vi "Begin.vi"(8 "error in":errorcluster) -> (0 "error out":errorcluster)   [LabVIEW 2015]
doc: "Called before other user functions, this VI is expected to open initial I/O refnums, load in file data, and do all program initialization. Notice that the <B>error out</B> terminal is simply used for data flow. Wiring it to other structures or subVIs ensures that this VI runs first."
uses:
  <vilib>/Rock Robotics/WPI/DriverStation/WPI_DriverStationRobotMode2.ctl
  <vilib>/Rock Robotics/WPI/Joystick/WPI_JoystickDeviceEnum.ctl
  <vilib>/Rock Robotics/SystemInterfaces/DIO/FPGA_DIOPWMChannel.ctl
  <vilib>/Rock Robotics/WPI/SafetyOutput/WPI_SafetyOutputConfigMenu.ctl
  <vilib>/Rock Robotics/SystemInterfaces/DIO/FPGA_DIOChannel.ctl
  <vilib>/Rock Robotics/WPI/Encoder/WPI_EncoderType.ctl
  <vilib>/Rock Robotics/WPI/CAN/TalonSRX/WPI_CANTalonSRX_APIControlMode.ctl
  <vilib>/Rock Robotics/WPI/CAN/TalonSRX/WPI_CANTalonSRX_APIFeedbackSelect.ctl
  Robot Global Data.vi
  <vilib>/Rock Robotics/Network Tables/NT Write String Array.vi
  <vilib>/Rock Robotics/WPI/RobotDrive/WPI_RobotDriveOpen2MotorWithTalon.vi
  <vilib>/Rock Robotics/WPI/Counter/WPI_CounterDigitalInputToDigitalSource.vi
  <vilib>/Rock Robotics/WPI/MotorControl/WPI_MotorControlOpenCANTalonSRX.vi
  <vilib>/Rock Robotics/WPI/RobotDrive/WPI_RobotDriveOpen2MotorWithJaguar.vi
panel:
  in  "I":dbl
  in  "F":dbl=0.01
  in  "D":dbl
  in  "P":dbl=1.0
  in  "Reverse Feedback Sensor":bool
  in  "Slave Device Number":u8=1
  in  "Encoder Codes Per Rev":u16=360
  in  "Master Device Number":u8
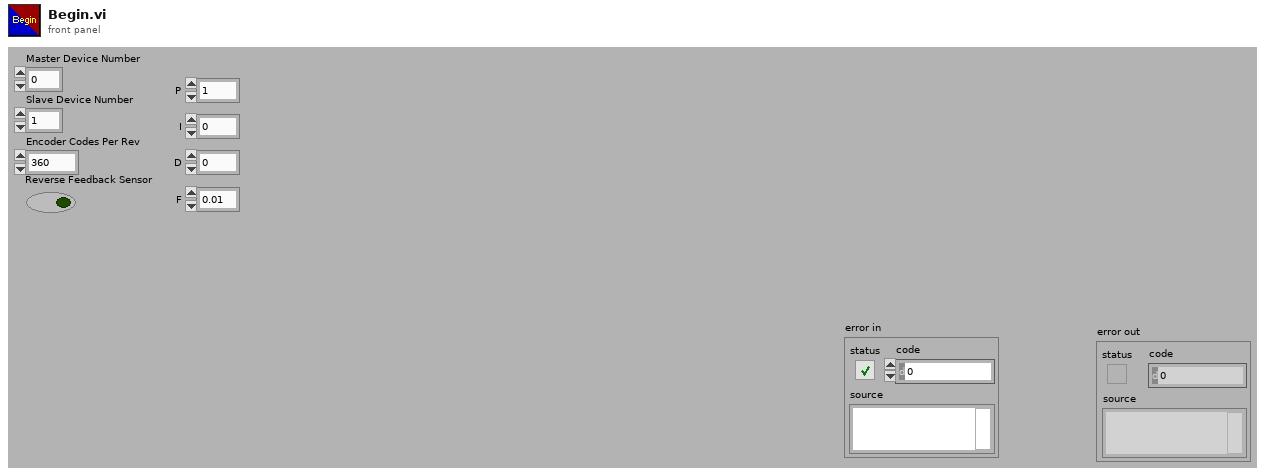
[diagram p1: front panel]
types:
  T1 = typedef "WPI_CANTalonSRX_APIControlMode.ctl" = enum8{"Percent VBus", "Speed", "Position", "Slave", "Unchanged / Invalid", "Voltage Compensation", "Current", "Motion Profile"}
  T2 = typedef "WPI_CANTalonSRX_APIFeedbackSelect.ctl" = enum16{"Digital Quadrature Encoder", "Analog Potentiometer", "Analog Encoder", "Count on Quad-A (Rising-Edge)", "Count on Quad-A (Falling-Edge)", "CTR Magnetic Enc (Absolute)", "CTR Magnetic Enc (Relative)", "Pulse Width"}
  T3 = typedef "WPI_EncoderType.ctl" = enum16{"1x", "2x", "4x"}
  T4 = typedef "FPGA_DIOChannel.ctl" = enum8{"DIO 0", "DIO 1", "DIO 2", "DIO 3", "DIO 4", "DIO 5", "DIO 6", "DIO 7", "DIO 8", "DIO 9", "DIO MXP 0", "DIO MXP 1", "DIO MXP 2", "DIO MXP 3", "DIO MXP 4", "DIO MXP 5", "DIO MXP 6", "DIO MXP 7", "DIO MXP 8", "DIO MXP 9", "DIO MXP 10", "DIO MXP 11", "DIO MXP 12", "DIO MXP 13", "DIO MXP 14", "DIO MXP 15", "Invalid"}
  T5 = typedef "FPGA_DIOPWMChannel.ctl" = enum8{"PWM 0", "PWM 1", "PWM 2", "PWM 3", "PWM 4", "PWM 5", "PWM 6", "PWM 7", "PWM 8", "PWM 9", "PWM MXP 0", "PWM MXP 1", "PWM MXP 2", "PWM MXP 3", "PWM MXP 4", "PWM MXP 5", "PWM MXP 6", "PWM MXP 7", "PWM MXP 8", "PWM MXP 9", "Invalid"}
  T6 = typedef "WPI_SafetyOutputConfigMenu.ctl" = enum16{"Enable", "Disable"}
  T7 = typedef "WPI_JoystickDeviceEnum.ctl" = enum16{"USB 0", "USB 1", "USB 2", "USB 3", "USB 4", "USB 5"}
  T8 = typedef "WPI_DriverStationRobotMode2.ctl" = enum16{"Autonomous Disabled", "Autonomous Enabled", "Teleop Disabled", "Teleop Enabled", "Disconnected", "Finish", "Test Disabled", "Test Enabled", "Emergency Stopped"}
  T9 = typedef "WPI_RobotDriveDevRef.ctl" = cluster{"DevStatus":errorcluster, "Motors[]":T10[], "Square Inputs":bool, "Max Output":dbl}
  T10 = typedef "WPI_MotorControlDeviceRef.ctl" = cluster{"DeviceStatus":errorcluster, "Type":T11, "PWM":cluster{"PWM Channel":T5, "DeadBand":T12}, "CAN":cluster{"Device Number":u8, "Control Mode":T13, "Semaphore":T14, "Max Vout":dbl, "TalonSRX Control Mode":T1}, "Invert":bool}
  T11 = typedef "WPI_MotorControlType.ctl" = enum16{"PWM", "CAN", "CANTalonSRX"}
  T12 = typedef "WPI_PWMDeadband.ctl" = cluster{"Name":string, "maxPositivePwm":i32, "minPositivePwm":i32, "centerPwm":i32, "maxNegativePwm":i32, "minNegativePwm":i32, "angularRange":u16}
  T13 = typedef "WPI_CANJaguar_ControlMode.ctl" = enum8{"Percent VBus", "Current", "Speed", "Position", "Voltage"}
  T14 = typedef "Semaphore RefNum" = refnum<k1>
  T15 = typedef "WPI_JoystickDevRef.ctl" = cluster{"Device":T7}
  T16 = typedef "WPI_DigitalInputDevRef.ctl" = cluster{"DevStatus":errorcluster, "DIO Channel":T4}
  T17 = typedef "FPGA_CounterEncoderSourceConvertionLVSourceType.ctl" = cluster{"DevStatus":errorcluster, "AnalogTriggerMode?":bool, "DigitalMode":cluster{"DIO Channel":T18}, "AnalogTriggerMode":cluster{"AnalogTriggerIndex":T19, "OutputType":T20}}
  T18 = typedef "FPGA_DIODigitalSourceChannel.ctl" = enum8{"DIO 0", "DIO 1", "DIO 2", "DIO 3", "DIO 4", "DIO 5", "DIO 6", "DIO 7", "DIO 8", "DIO 9", "DIO MXP 0", "DIO MXP 1", "DIO MXP 2", "DIO MXP 3", "DIO MXP 4", "DIO MXP 5", "DIO MXP 6", "DIO MXP 7", "DIO MXP 8", "DIO MXP 9", "DIO MXP 10", "DIO MXP 11", "DIO MXP 12", "DIO MXP 13", "DIO MXP 14", "DIO MXP 15", "Disabled"}
  T19 = typedef "FPGA_AnalogTriggerIndex.ctl" = enum8{"Trig 0", "Trig 1", "Trig 2", "Trig 3", "Trig 4", "Trig 5", "Trig 6", "Trig 7", "Invalid"}
  T20 = typedef "FPGA_AnalogTriggerOutType.ctl" = enum16{"InWindow", "TriggerState", "Rising", "Falling"}
  T21 = typedef "WPI_EncoderDevRef.ctl" = cluster{"DevStatus":errorcluster, "EncoderIndex":T22, "CounterIndex":T23, "DistancePerCount":dbl, "Decoding Type":T3}
  T22 = typedef "FPGA_EncoderIdx.ctl" = enum8{"Enc 0", "Enc 1", "Enc 2", "Enc 3", "Enc 4", "Enc 5", "Enc 6", "Enc 7", "Invalid"}
  T23 = typedef "FPGA_CounterCtrSystemIndex.ctl" = enum8{"Ctr 0", "Ctr 1", "Ctr 2", "Ctr 3", "Ctr 4", "Ctr 5", "Ctr 6", "Ctr 7", "Invalid"}
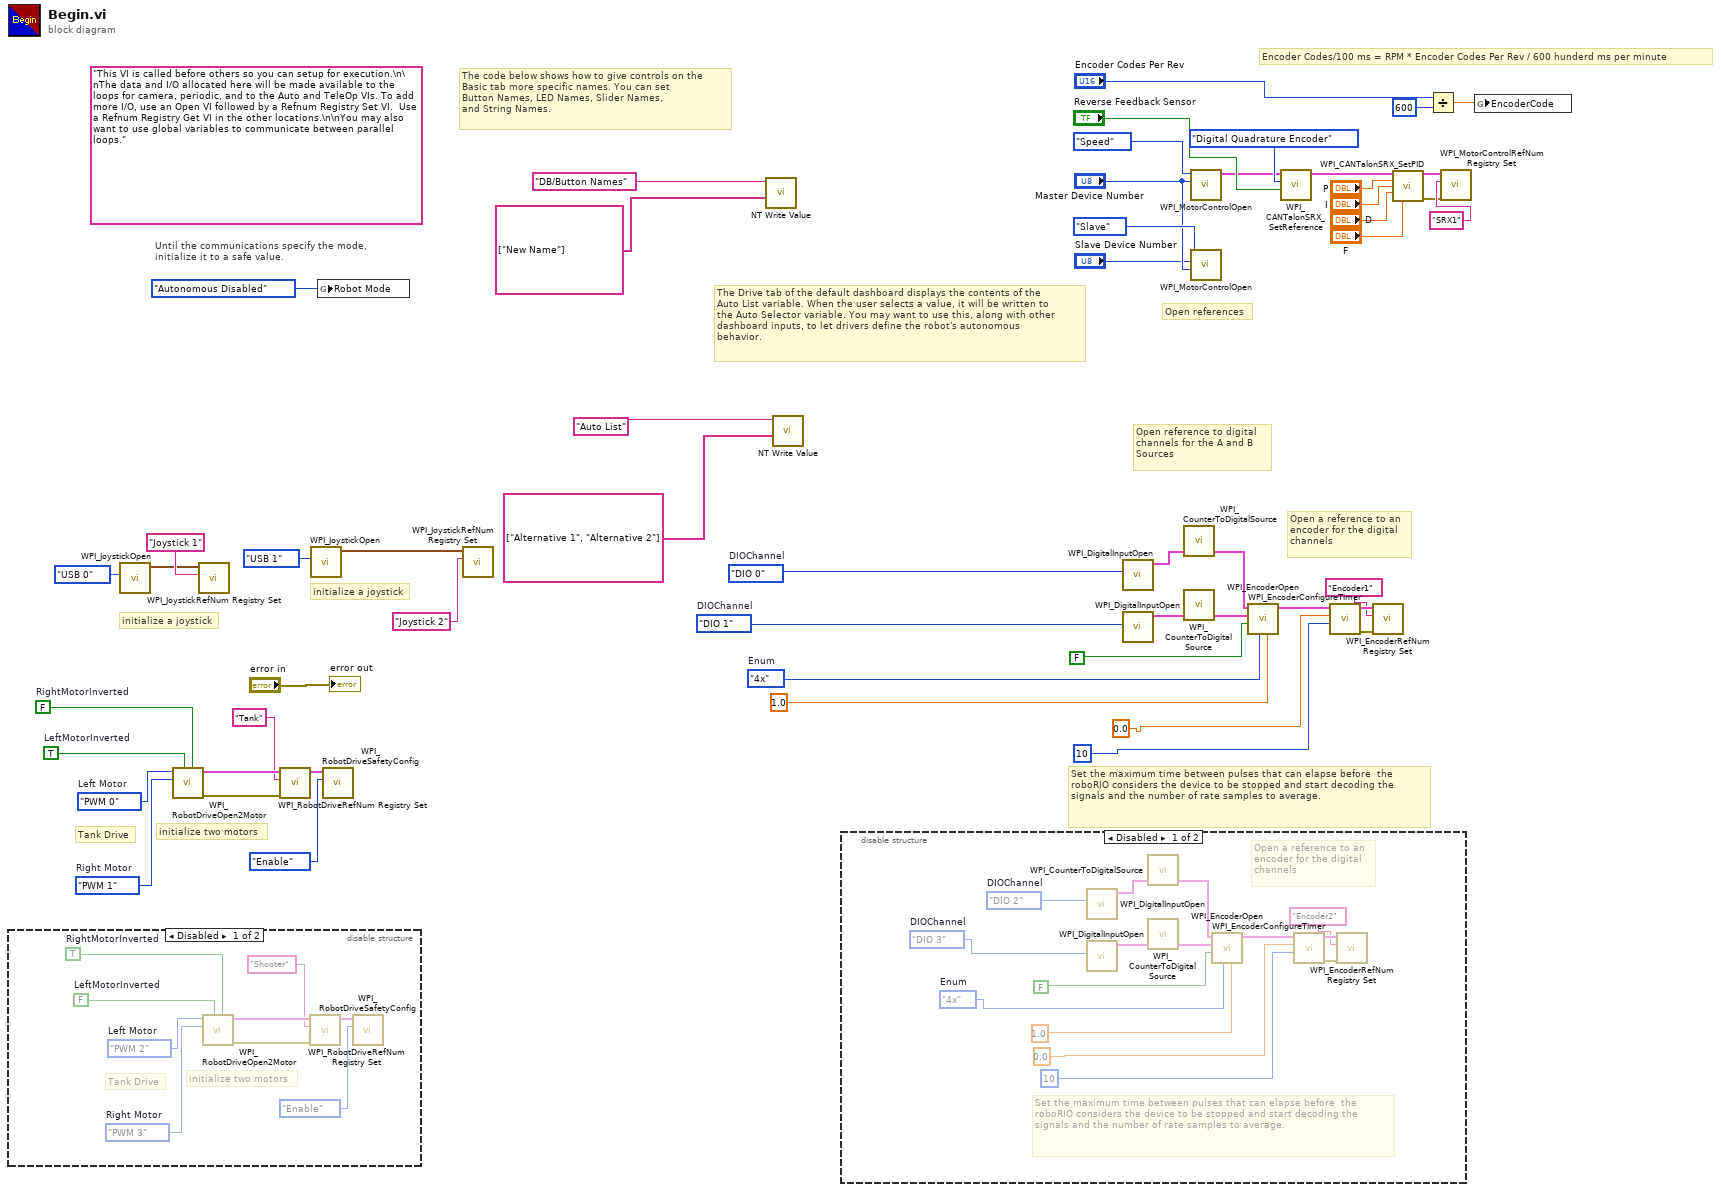
[diagram p0: block diagram]
diagram:
  w22 = WPI_EncoderType."4x"  # Enum
  w24 = FPGA_DIOChannel."DIO 1"  # DIOChannel
  w25 = FPGA_DIOChannel."DIO 0"  # DIOChannel
  w34 = FPGA_DIOPWMChannel."PWM 1"  # Right Motor
  w37 = FPGA_DIOPWMChannel."PWM 0"  # Left Motor
  w41 = TRUE  # LeftMotorInverted
  w42 = FALSE  # RightMotorInverted
  (unwired) "This VI is called before others so you can setup for execution.\n\nThe data and I/O allocated here will be made available to the loops for camera, periodic, and to the Auto and TeleOp VIs. To add more I/O, use an Open VI followed by a Refnum Registry Set VI.  Use a Refnum Registry Get VI in the other locations.\n\nYou may also want to use global variables to communicate between parallel loops."
  # "Encoder Codes/100 ms = RPM * Encoder Codes Per Rev / 600 hunderd ms per minute"
  # "Open references"
  # "The Drive tab of the default dashboard displays the contents of the\nAuto List variable. When the user selects a value, it will be written to\nthe Auto Selector variable. You may want to use this, along with other\ndashboard inputs, to let drivers define the robot's autonomous\nbehavior."
  # "Set the maximum time between pulses that can elapse before  the roboRIO considers the device to be stopped and start decoding the signals and the number of rate samples to average."
  # "Open a reference to an\nencoder for the digital \nchannels"
  # "Tank Drive"
  # "initialize two motors"
  # "Open reference to digital \nchannels for the A and B\nSources"
  # "initialize a joystick"
  # "initialize a joystick"
  # "The code below shows how to give controls on the\nBasic tab more specific names. You can set\nButton Names, LED Names, Slider Names,\nand String Names."
  # "Until the communications specify the mode,\ninitialize it to a safe value."
  n1 = disable-structure shown="Disabled" {
    frame Disabled {
      w55 = FPGA_DIOPWMChannel."PWM 3"  # Right Motor
      w58 = FPGA_DIOPWMChannel."PWM 2"  # Left Motor
      w62 = FALSE  # LeftMotorInverted
      w63 = TRUE  # RightMotorInverted
      # "Tank Drive"
      # "initialize two motors"
      n2 = call-poly <vilib>:"WPI_RobotDriveOpen2Motor.vi"("Right Motor Inverted"=w63, "Left Motor Inverted"=w62, "Right Motor"=w55, "Left Motor"=w58) -> ("error out"=w59:errorcluster, "RobotDriveDevRef"=w61:T9)  [unwired: 1 in, 5 out]
      n3 = call <vilib>:"WPI_RobotDriveRefNum Registry Set.vi"("error in (no error)"=w59, "refnum name"="Shooter", "RobotDriveDevRef"=w61) -> ("RobotDriveDevRef"=w57:T9)  [unwired: 1 in, 7 out]
      n4 = call <vilib>:"WPI_RobotDriveSafetyConfig.vi"("mode"=WPI_SafetyOutputConfigMenu."Enable", "RobotDriveDevRef"=w57) -> ()  [unwired: 8 in, 2 out]
    }
    frame Enabled {
    }
  }
  n5 = call <vilib>:"WPI_JoystickOpen.vi"("JoystickDevice"=WPI_JoystickDeviceEnum."USB 0") -> ("JoystickDevRef"=w47:T15)  [unwired: 10 in]
  n6 = call-poly <vilib>:"WPI_RobotDriveOpen2Motor.vi"("Right Motor Inverted"=w42, "Left Motor Inverted"=w41, "Right Motor"=w34, "Left Motor"=w37) -> ("error out"=w38:errorcluster, "RobotDriveDevRef"=w40:T9)  [unwired: 1 in, 5 out]
  n7 = call <vilib>:"WPI_JoystickRefNum Registry Set.vi"("refnum name"="Joystick 1", "JoystickDevRef"=w47) -> ()  [unwired: 8 in, 2 out]
  n8 = call <vilib>:"WPI_RobotDriveRefNum Registry Set.vi"("error in (no error)"=w38, "refnum name"="Tank", "RobotDriveDevRef"=w40) -> ("RobotDriveDevRef"=w36:T9)  [unwired: 1 in, 7 out]
  n9 = call <vilib>:"WPI_JoystickOpen.vi"("JoystickDevice"=WPI_JoystickDeviceEnum."USB 1") -> ("JoystickDevRef"=w44:T15)  [unwired: 10 in]
  n10 = global write "Robot Global Data.vi" "Robot Mode"(WPI_DriverStationRobotMode2."Autonomous Disabled" ("Robot Mode")) -> ()
  n11 = call <vilib>:"WPI_RobotDriveSafetyConfig.vi"("mode"=WPI_SafetyOutputConfigMenu."Enable", "RobotDriveDevRef"=w36) -> ()  [unwired: 8 in, 2 out]
  n12 = call <vilib>:"WPI_JoystickRefNum Registry Set.vi"("refnum name"="Joystick 2", "JoystickDevRef"=w44) -> ()  [unwired: 8 in, 2 out]
  n13 = call-poly <vilib>:"NT Write Value.vi"("String Array"=string[] ["New Name"], "Name"="DB/Button Names") -> ()  [unwired: 9 in, 1 out]
  n14 = call-poly <vilib>:"NT Write Value.vi"("String Array"=string[] ["Alternative 1", "Alternative 2"], "Name"="Auto List") -> ()  [unwired: 9 in, 1 out]
  n15 = disable-structure shown="Disabled" {
    frame Disabled {
      w67 = WPI_EncoderType."4x"  # Enum
      w69 = FPGA_DIOChannel."DIO 3"  # DIOChannel
      w70 = FPGA_DIOChannel."DIO 2"  # DIOChannel
      # "Set the maximum time between pulses that can elapse before  the roboRIO considers the device to be stopped and start decoding the signals and the number of rate samples to average."
      # "Open a reference to an\nencoder for the digital \nchannels"
      n16 = call <vilib>:"WPI_DigitalInputOpen.vi"("DIO Channel"=w70) -> ("DigitalInputDevRef"=w76:T16)  [unwired: 1 in, 9 out]
      n17 = call <vilib>:"WPI_DigitalInputOpen.vi"("DIO Channel"=w69) -> ("DigitalInputDevRef"=w77:T16)  [unwired: 1 in, 9 out]
      n18 = call-poly <vilib>:"WPI_CounterToDigitalSource.vi"("DigitalInputDevRef"=w76) -> ("Digital Source"=w75:T17)  [unwired: 6 out]
      n19 = call-poly <vilib>:"WPI_CounterToDigitalSource.vi"("DigitalInputDevRef"=w77) -> ("Digital Source"=w78:T17)  [unwired: 6 out]
      n20 = call <vilib>:"WPI_EncoderOpen.vi"("DistancePerCount"=1.0, "Decoding Type"=w67, "Invert Direction (False)"=FALSE, "BSource"=w78, "ASource"=w75) -> ("EncoderDevRef"=w74:T21)  [unwired: 3 in, 3 out]
      n21 = call <vilib>:"WPI_EncoderConfigureTimer.vi"("Number Samples to Average"=10, "Minimum Rate"=0.0, "EncoderDevRef"=w74) -> ("error out"=w73:errorcluster, "EncoderDevRef"=w72:T21)  [unwired: 1 in, 6 out]
      n22 = call <vilib>:"WPI_EncoderRefNum Registry Set.vi"("error in (no error)"=w73, "refnum name"="Encoder2", "EncoderDevRef"=w72) -> ()  [unwired: 7 in, 2 out]
    }
    frame Enabled {
    }
  }
  n23 = call <vilib>:"WPI_DigitalInputOpen.vi"("DIO Channel"=w25) -> ("DigitalInputDevRef"=w31:T16)  [unwired: 1 in, 9 out]
  n24 = call <vilib>:"WPI_DigitalInputOpen.vi"("DIO Channel"=w24) -> ("DigitalInputDevRef"=w32:T16)  [unwired: 1 in, 9 out]
  n25 = call-poly <vilib>:"WPI_CounterToDigitalSource.vi"("DigitalInputDevRef"=w31) -> ("Digital Source"=w30:T17)  [unwired: 6 out]
  n26 = call-poly <vilib>:"WPI_CounterToDigitalSource.vi"("DigitalInputDevRef"=w32) -> ("Digital Source"=w33:T17)  [unwired: 6 out]
  n27 = call-poly <vilib>:"WPI_MotorControlOpen.vi"("Device Number"="Master Device Number", "Control Mode"=WPI_CANTalonSRX_APIControlMode."Speed") -> ("MotorControlDeviceRef"=w8:T10)  [unwired: 3 in, 6 out]
  n28 = call-poly <vilib>:"WPI_MotorControlOpen.vi"("Master Device Number"="Master Device Number", "Device Number"="Slave Device Number", "Control Mode"=WPI_CANTalonSRX_APIControlMode."Slave") -> ()  [unwired: 2 in, 7 out]
  n29 = call <vilib>:"WPI_EncoderOpen.vi"("DistancePerCount"=1.0, "Decoding Type"=w22, "Invert Direction (False)"=FALSE, "BSource"=w33, "ASource"=w30) -> ("EncoderDevRef"=w29:T21)  [unwired: 3 in, 3 out]
  n30 = call <vilib>:"WPI_CANTalonSRX_SetReference.vi"("Reverse Feedback Sensor"="Reverse Feedback Sensor", "Feedback Reference"=WPI_CANTalonSRX_APIFeedbackSelect."Digital Quadrature Encoder", "CAN Talon SRX Ref"=w8) -> ("CAN Talon SRX Ref"=w7:T10)  [unwired: 7 in, 1 out]
  n31 = call <vilib>:"WPI_EncoderConfigureTimer.vi"("Number Samples to Average"=10, "Minimum Rate"=0.0, "EncoderDevRef"=w29) -> ("error out"=w28:errorcluster, "EncoderDevRef"=w27:T21)  [unwired: 1 in, 6 out]
  n32 = call <vilib>:"WPI_EncoderRefNum Registry Set.vi"("error in (no error)"=w28, "refnum name"="Encoder1", "EncoderDevRef"=w27) -> ()  [unwired: 7 in, 2 out]
  n33 = call <vilib>:"WPI_CANTalonSRX_SetPID.vi"("CAN Talon SRX Ref"=w7, "P"="P", "I"="I", "D"="D", "F"="F") -> ("CAN Talon SRX Ref"=w3:T10, "error out"=w1:errorcluster)  [unwired: 9 in]
  n34 = Divide(x="Encoder Codes Per Rev", y=u16 600) -> (x/y=w4:dbl)
  n35 = call <vilib>:"WPI_MotorControlRefNum Registry Set.vi"("error in (no error)"=w1, "refnum name"="SRX1", "MotorControlDevRef"=w3) -> ()  [unwired: 7 in, 2 out]
  n36 = global write "Robot Global Data.vi" "EncoderCode"(w4) -> ()
  "error out" <- "error in"
